vi "SubVI_Example_Has_PixelClockRange.vi"(0 ".NET (Reference)":refnum<k24>, 5 "error in (no error)":errorcluster) -> (14 "Boolean":bool, 19 "error out":errorcluster)   [LabVIEW 2016]
uses:
  C:/Program Files/National Instruments/LabVIEW 2016/instr.lib/IDS/ueye.NET/uEyeDotNet.dll
  Program Files/National Instruments/LabVIEW 2016/instr.lib/IDS/ueye.NET/uEyeDotNet.dll
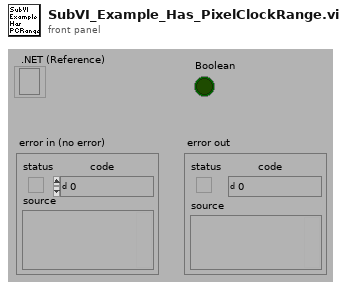
[diagram p1: front panel]
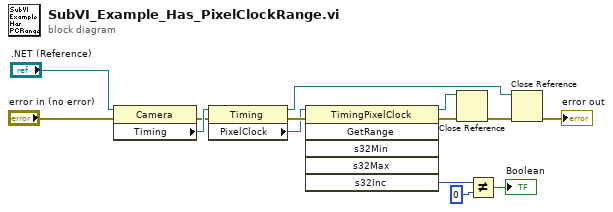
[diagram p0: block diagram]
diagram:
  n1 = property class="Camera"(reference=".NET (Reference)", error in="error in (no error)") -> (error out=w11:errorcluster, "Timing"=w12:refnum<k24>)  [unwired: 1 out]
  n2 = property class="Timing"(reference=w12, error in=w11) -> (reference out=w8:refnum<k24>, error out=w10:errorcluster, "PixelClock"=w9:refnum<k24>)
  n3 = invoke class="TimingPixelClock" method="GetRange"(reference=w9, error in=w10) -> (reference out=w3:refnum<k24>, error out=w2:errorcluster, "s32Inc"=w4:i32)  [unwired: 4 in, 3 out]
  n4 = Close Reference(reference=w3, error in (no error)=w2) -> (error out=w1:errorcluster)
  n5 = Not Equal?(x=w4, y=0) -> (x != y?=→"Boolean":bool)
  n6 = Close Reference(reference=w8, error in (no error)=w1) -> (error out=→"error out":errorcluster)
